vi "Configure 2 Wire Resistance.vi"(0 "VISA resource name":refnum<visa-resource-name>, 1 "Resolution (7: 6.5 digits)":u16(ring)=7 items=["3.5 Digits"=4, "4.5 Digits"=5, "5.5 Digits"=6, "6.5 Digits"=7], 2 "Power Line Cycles (1.00)":dbl=1.0 format="%.2f", 5 "error in (no error)":errorcluster, 6 "Auto Range? (T: Auto)":bool=TRUE, 7 "Digital Filter (0: Off)":u16(ring) items=["Off", "Moving Filter", "Repeating Filter"], 8 "Custom Range (0 Ohm)":dbl format="%#_6p", 9 "Digital Filter Readings (10)":i32=10, 10 "Reference (0: Off)":u16(ring) items=["Off", "Set", "Acquire"], 12 "Reference Value (0.000 Ohm)":dbl format="%_3g") -> (14 "VISA resource name out":refnum<visa-resource-name>, 19 "error out":errorcluster)   [LabVIEW 2013, in "Keithley 2000.lvlib"]
doc: "This VI configures the instrument to measure 2-Wire Resistance.\n\nNote:\nWhen reading measurements (using the \"Data Read Single\" or \"Data Read Multiple\" VIs), a value of 9.9E+37 indicates overflow (i.e., an open circuit)."
uses:
  Keithley 2000.lvlib
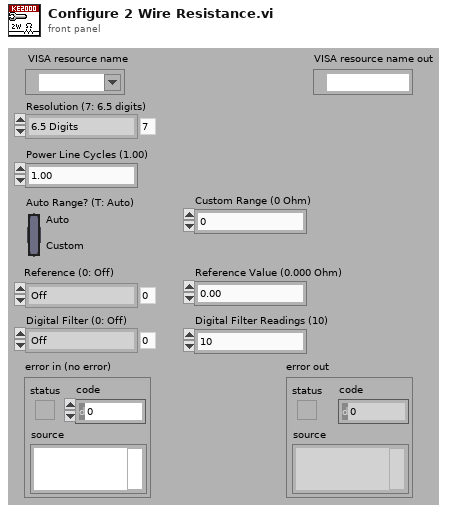
[diagram p1: front panel]
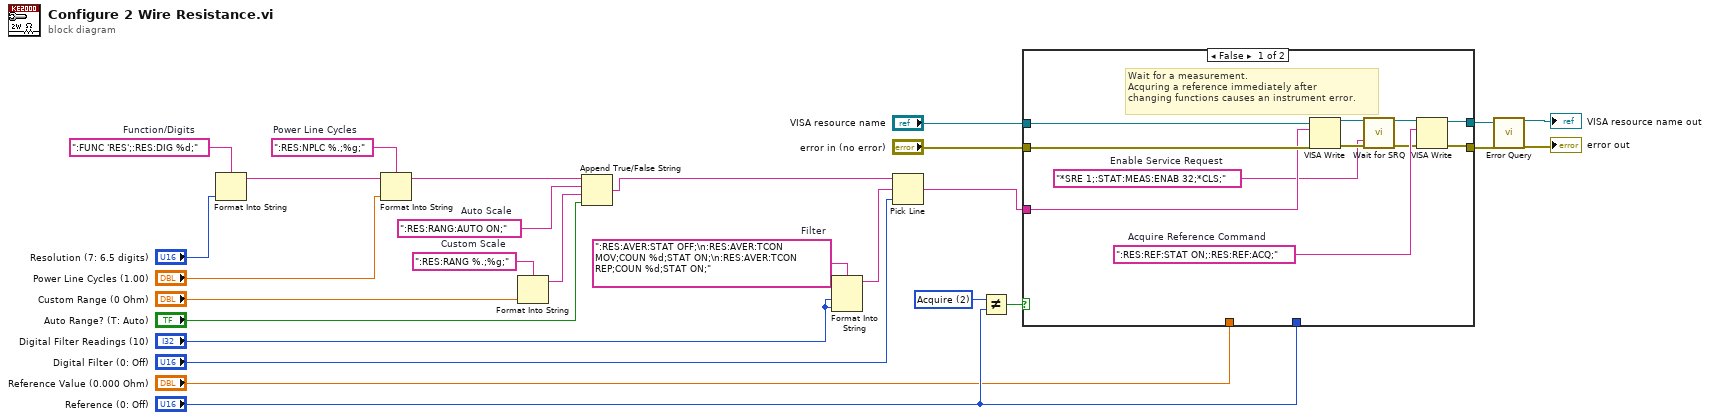
[diagram p0: block diagram]
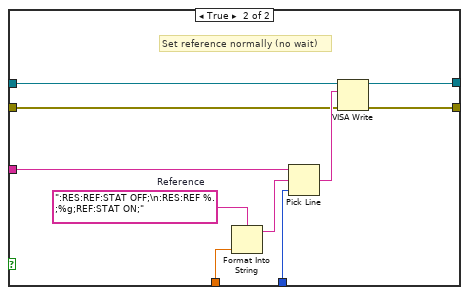
[diagram p2: hidden frame]
diagram:
  w9 = u16 2 items=["Off", "Set", "Acquire"] ("Reference (0: Off)")
  w14 = ":RES:NPLC %.;%g;"  # Power Line Cycles
  w16 = ":RES:AVER:STAT OFF;\n:RES:AVER:TCON MOV;COUN %d;STAT ON;\n:RES:AVER:TCON REP;COUN %d;STAT ON;"  # Filter
  w19 = ":RES:RANG:AUTO ON;"  # Auto Scale
  w21 = ":RES:RANG %.;%g;"  # Custom Scale
  w22 = ":FUNC 'RES';:RES:DIG %d;"  # Function/Digits
  n1 = Format Into String(format string=w22, "Resolution (7: 6.5 digits)") -> (resulting string=w13:string)  [unwired: 2 in, 1 out]
  n2 = Format Into String(format string=w14, initial string=w13, "Power Line Cycles (1.00)") -> (resulting string=w24:string)  [unwired: 1 in, 1 out]
  n3 = Format Into String(format string=w21, "Custom Range (0 Ohm)") -> (resulting string=w20:string)  [unwired: 2 in, 1 out]
  n4 = Append True/False String(1:"Auto Range? (T: Auto)", 2:w20, 3:w19, 4:w24) -> (0:w10:string)
  n5 = Format Into String(format string=w16, "Digital Filter Readings (10)", "Digital Filter Readings (10)") -> (resulting string=w17:string)  [unwired: 2 in, 1 out]
  n6 = Pick Line(string ("")=w10, multi-line string=w17, line index="Digital Filter (0: Off)") -> (output string=w3:string)
  n7 = Not Equal?(x=w9, y="Reference (0: Off)") -> (x != y?=w6:bool)
  n8 = case shown="False" w6 {
    tunnel: "VISA resource name" -> [w35 w41]
    tunnel: "error in (no error)" -> [w36 w40]
    tunnel: "Reference Value (0.000 Ohm)" -> [_ w46]
    tunnel: w3 -> [w29 w39]
    tunnel: [w30 w45] -> w2
    tunnel: [w31 w44] -> w1
    tunnel: "Reference (0: Off)" -> [_ w42]
    frame False {
      w28 = "*SRE 1;:STAT:MEAS:ENAB 32;*CLS;"  # Enable Service Request
      w34 = ":RES:REF:STAT ON;:RES:REF:ACQ;"  # Acquire Reference Command
      # "Wait for a measurement.\nAcquring a reference immediately after\nchanging functions causes an instrument error."
      n9 = VISA Write(VISA resource name=w35, write buffer=w29, error in (no error)=w36) -> (VISA resource name out=w38:refnum<visa-resource-name>, error out=w37:errorcluster)  [unwired: 1 out]
      n10 = call "Wait for SRQ.vi"("VISA resource name"=w38, "SRQ Enable Command"=w28, "error in (no error)"=w37) -> ("VISA resource name out"=w33:refnum<visa-resource-name>, "error out"=w32:errorcluster)  [unwired: 15 in]
      n11 = VISA Write(VISA resource name=w33, write buffer=w34, error in (no error)=w32) -> (VISA resource name out=w31:refnum<visa-resource-name>, error out=w30:errorcluster)  [unwired: 1 out]
    }
    frame True {
      w48 = ":RES:REF:STAT OFF;\n:RES:REF %.;%g;REF:STAT ON;"  # Reference
      # "Set reference normally (no wait)"
      n12 = Format Into String(format string=w48, w46) -> (resulting string=w47:string)  [unwired: 2 in, 1 out]
      n13 = Pick Line(string ("")=w39, multi-line string=w47, line index=w42) -> (output string=w43:string)
      n14 = VISA Write(VISA resource name=w41, write buffer=w43, error in (no error)=w40) -> (VISA resource name out=w44:refnum<visa-resource-name>, error out=w45:errorcluster)  [unwired: 1 out]
    }
  }
  n15 = call "Error Query.vi"("VISA resource name"=w1, "error in (no error)"=w2) -> ("VISA resource name out"=→"VISA resource name out":refnum<visa-resource-name>, "error out"=→"error out":errorcluster)  [unwired: 14 in, 2 out]
